vi "nirvimemoryEmulation.vi"(0 "Address":u32, 1 "Name":string, 2 "Depth":i32, 3 "Initialization Data":variant[](array[variant]), 5 "Data":i32, 7 "Write? (F)":bool, 9 "inTimedLoop":bool, 11 "error in":errorcluster, 12 "Local? (F)":bool, 13 "ref in wired":bool) -> (6 "Data":i32, 15 "error out":errorcluster)   [LabVIEW 2017]
uses:
  <vilib>/rvi/Emulation/niFpgaSctlEmulationSharedResMgrCmd.ctl
  <vilib>/rvi/Emulation/niFpgaSctlEmulationSharedResource.ctl
  <vilib>/rvi/Emulation/niFpgaSctlEmulationSharedResTypes.ctl
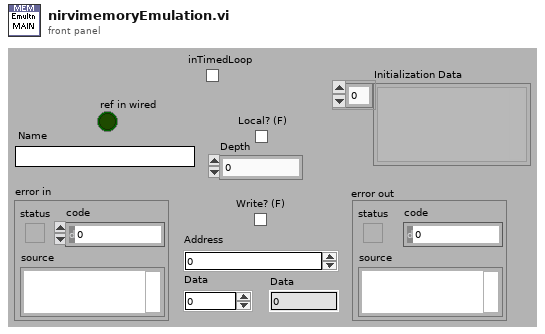
[diagram p1: front panel]
types:
  T1 = typedef "niFpgaSctlEmulationSharedResTypes.ctl" = enum16{"Global", "Register", "Fifo", "Full Memory", "Fast Memory", "Local"}
  T2 = typedef "niFpgaSctlEmulationSharedResource.ctl" = cluster{"resourceType":T1, "dataToWrite":variant, "ref":u32, "index":i32, "resourceName":string}
  T3 = typedef "niFpgaSctlEmulationSharedResMgrCmd.ctl" = enum16{"UpdateResources", "AddResource"}
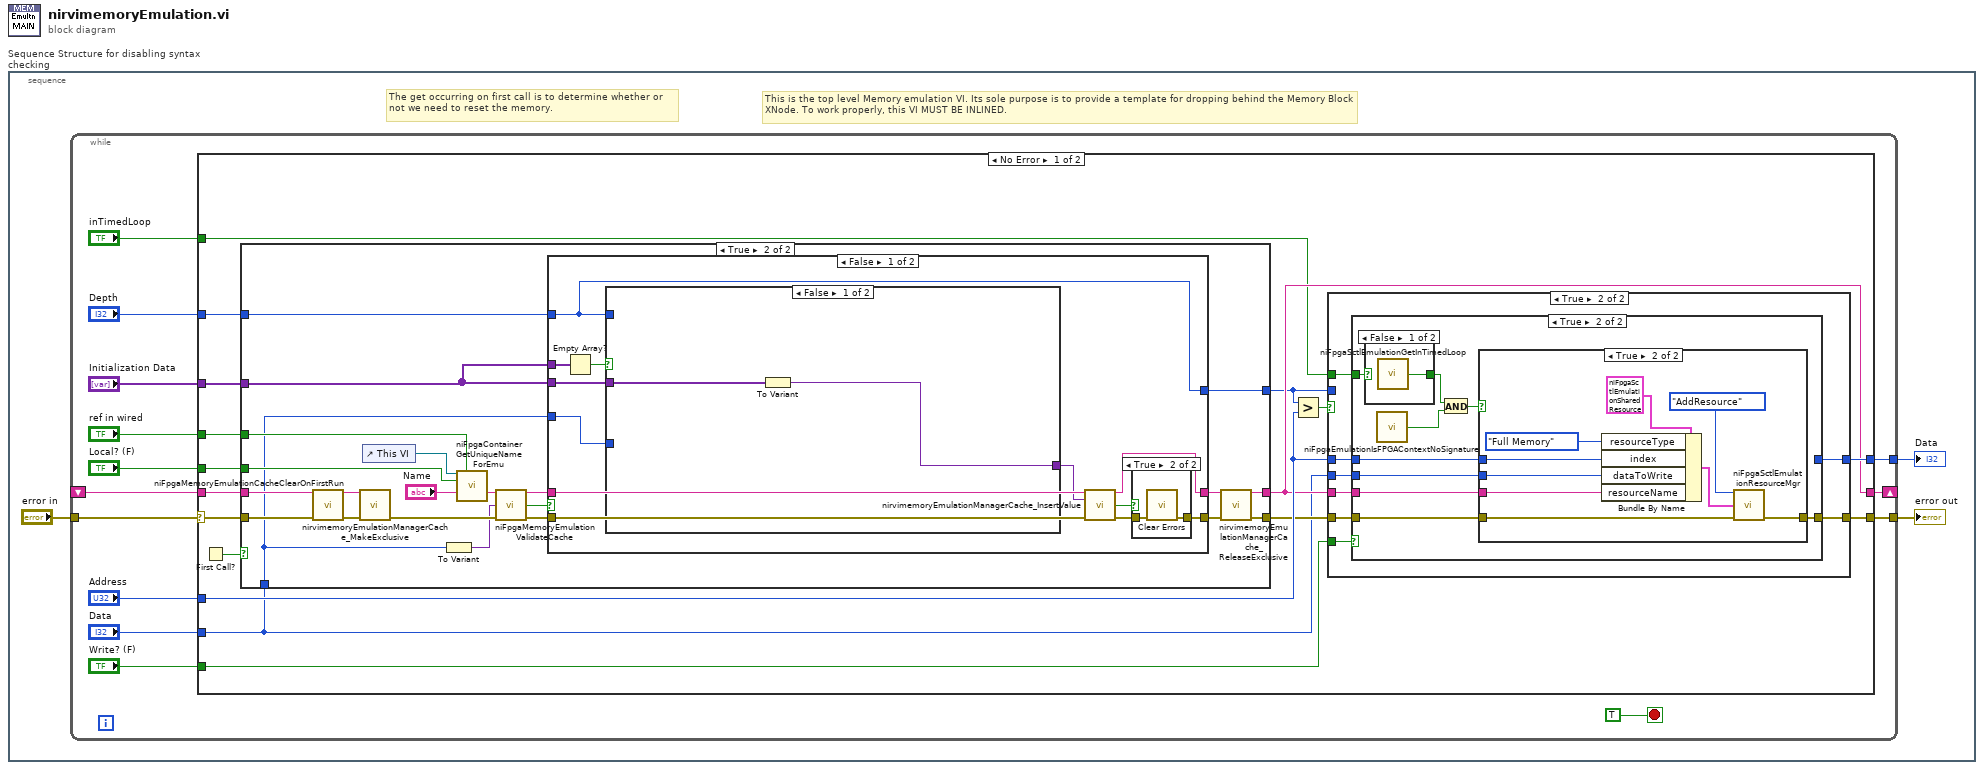
[diagram p0: block diagram]
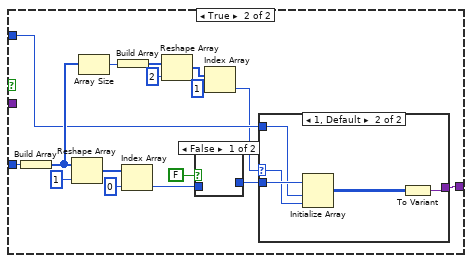
[diagram p3: hidden frame]
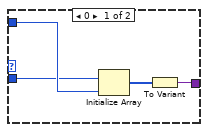
[diagram p4: hidden frame]
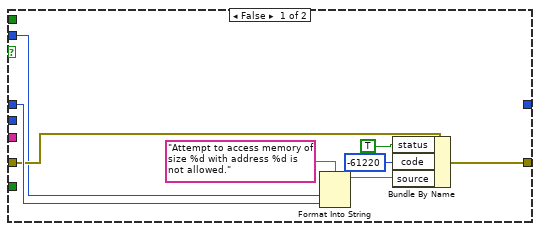
[diagram p8: hidden frame]
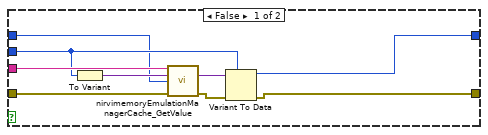
[diagram p9: hidden frame]
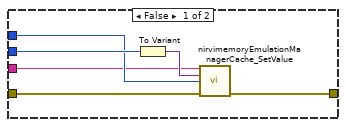
[diagram p11: hidden frame]
diagram:
  n1 = stacked-sequence "Sequence Structure for disabling syntax checking" {
    frame #0 {
      # "The get occurring on first call is to determine whether or not we need to reset the memory."
      # "This is the top level Memory emulation VI. Its sole purpose is to provide a template for dropping behind the Memory Block XNode. To work properly, this VI MUST BE INLINED."
      n2 = while {
        shift-right: [w15] -> _
        shift-left: _ -> [w17]
        tunnel: [w14] -> w1
        tunnel: [w13] -> w2
        tunnel: "error in" -> [w8]
        stop <- TRUE stop-if-true
        n3 = case shown="No Error" w8 {
          selector: w8 -> [w27 w158]
          tunnel: "Depth" -> [w25 _]
          tunnel: w17 -> [w26 w157]
          tunnel: [w29 w157] -> w15
          tunnel: "Write? (F)" -> [w32 _]
          tunnel: [w31 w158] -> w14
          tunnel: "Address" -> [w33 _]
          tunnel: "Data" -> [w24 _]
          tunnel: [w30 _] -> w13
          tunnel: "ref in wired" -> [w23 _]
          tunnel: "Local? (F)" -> [w22 _]
          tunnel: "inTimedLoop" -> [w19 _]
          tunnel: "Initialization Data" -> [w18 _]
          frame No Error {
            n4 = First Call?() -> (First Call?: T/F=w20:bool)
            n5 = case shown="True" w20 {
              tunnel: [w37 w59] -> w29
              tunnel: [w36 w58] -> w28
              tunnel: w27 -> [w36 w56]
              tunnel: w26 -> [w37 w55]
              tunnel: w25 -> [w35 w54]
              tunnel: w24 -> [_ w39]
              tunnel: w23 -> [_ w53]
              tunnel: w22 -> [_ w52]
              tunnel: [w35 w51] -> w21
              tunnel: w18 -> [_ w38]
              frame False {
              }
              frame True {
                n6 = call <vilib>:"niFpgaMemoryEmulationCacheClearOnFirstRun.vi"("Key"=w55, "error in"=w56) -> ("Key (dup)"=w50:string, "error out"=w57:errorcluster)  [unwired: 12 in]
                n7 = call <vilib>:"nirvimemoryEmulationManagerCache_MakeExclusive.vi"("Key"=w50, "error in"=w57) -> ("error out"=w41:errorcluster)  [unwired: 12 in, 1 out]
                n8 = control-ref of="This VI"() -> (w42:refnum<vi>)
                n9 = To Variant(anything=w39) -> (Variant=w40:variant)
                n10 = call <vilib>:"niFpgaContainerGetUniqueNameForEmu.vi"("parent VI"=w42, "ref in wired"=w53, "local"=w52, "name in"="Name") -> ("name out"=w44:string)  [unwired: 11 in]
                n11 = call <vilib>:"niFpgaMemoryEmulationValidateCache.vi"("key"=w44, "Data In"=w40, "error in"=w41) -> ("key (dup)"=w49:string, "found?"=w47:bool, "error out"=w48:errorcluster)  [unwired: 10 in]
                n12 = case shown="False" w47 {
                  tunnel: [w69 w105] -> w46
                  tunnel: [w60 w104] -> w51
                  tunnel: [w68 w103] -> w45
                  tunnel: w54 -> [w60 w104]
                  tunnel: w49 -> [w66 w105]
                  tunnel: w48 -> [w67 w103]
                  tunnel: w38 -> [w63 _]
                  tunnel: w38 -> [w62 _]
                  tunnel: w39 -> [w61 _]
                  frame False {
                    n13 = Empty Array?(array=w63) -> (empty?=w65:bool)
                    n14 = case shown="False" w65 {
                      tunnel: [w72 w74] -> w64
                      tunnel: w62 -> [w73 _]
                      tunnel: w61 -> [_ w80]
                      tunnel: w60 -> [_ w77]
                      frame False {
                        n15 = To Variant(anything=w73) -> (Variant=w72:variant)
                      }
                      frame True {
                        n16 = Build Array(w80) -> (w89:i32[])
                        n17 = Reshape Array(w89, 1 ("dimension size")) -> (w81:i32[])
                        n18 = Array Size(array=w89) -> (size(s)=w88:i32)
                        n19 = Build Array(w88) -> (w86:i32[])
                        n20 = Index Array(array=w81, index=0) -> (element=w76:i32)
                        n21 = Reshape Array(w86, 2 ("dimension size")) -> (w84:i32[])
                        n22 = case shown="False" FALSE {
                          tunnel: w76 -> [_ w99]
                          tunnel: [_ w99] -> w79
                          frame False {
                          }
                          frame True {
                          }
                        }
                        n23 = Index Array(array=w84, index=1) -> (element=w75:i32)
                        n24 = case shown="1, Default" w75 {
                          selector: w75 -> [_ w94]
                          tunnel: w79 -> [w91 w97]
                          tunnel: w77 -> [w92 w95]
                          tunnel: [w93 w98] -> w74
                          frame 0 {
                            n25 = Initialize Array(w91, w92) -> (w90:i32[])
                            n26 = To Variant(anything=w90) -> (Variant=w93:variant)
                          }
                          frame 1, Default {
                            n27 = Initialize Array(w97, w95, w94) -> (w96:i32[][])
                            n28 = To Variant(anything=w96) -> (Variant=w98:variant)
                          }
                        }
                      }
                    }
                    n29 = call <vilib>:"nirvimemoryEmulationManagerCache_InsertValue.vi"("Key"=w66, "Value"=w64, "error in (no error)"=w67) -> ("Key"=w69:string, "Found"=w71:bool, "error out"=w70:errorcluster)  [unwired: 1 in, 9 out]
                    n30 = case shown="True" w71 {
                      tunnel: w70 -> [w100 w102]
                      tunnel: [w100 w101] -> w68
                      frame False {
                      }
                      frame True {
                        n31 = call <vilib>:"Clear Errors.vi"("error in (no error)"=w102) -> ("error out"=w101:errorcluster)  [unwired: 1 in, 5 out]
                      }
                    }
                  }
                  frame True {
                  }
                }
                n32 = call <vilib>:"nirvimemoryEmulationManagerCache_ReleaseExclusive.vi"("Key"=w46, "error in"=w45) -> ("Key (dup)"=w59:string, "error out"=w58:errorcluster)  [unwired: 12 in]
              }
            }
            n33 = Greater?(x=w21, y=w33) -> (0:w34:bool)
            n34 = case shown="True" w34 {
              tunnel: w24 -> [_ w116]
              tunnel: w33 -> [w113 w119]
              tunnel: w28 -> [w112 w117]
              tunnel: w29 -> [_ w118]
              tunnel: w32 -> [_ w115]
              tunnel: [w111 w121] -> w31
              tunnel: [_ w120] -> w30
              tunnel: w21 -> [w107 _]
              tunnel: w19 -> [_ w114]
              frame False {
                n35 = Format Into String(format string="Attempt to access memory of size %d with address %d is not allowed." ("error message (\"\")"), w107, w113) -> (resulting string=w108:string)  [unwired: 2 in, 1 out]
                n36 = Bundle By Name(cluster=w112, "status"=TRUE, "code"=-61220, "source"=w108) -> (w111:errorcluster)
              }
              frame True {
                n37 = case shown="True" w115 {
                  tunnel: [w130 w135] -> w121
                  tunnel: [w123 _] -> w120
                  tunnel: w119 -> [w122 w139]
                  tunnel: w118 -> [w127 w136]
                  tunnel: w117 -> [w126 w137]
                  tunnel: w116 -> [w124 w138]
                  tunnel: w114 -> [_ w134]
                  frame False {
                    n38 = To Variant(anything=w124) -> (Variant=w125:variant)
                    n39 = call <vilib>:"nirvimemoryEmulationManagerCache_GetValue.vi"("Key"=w127, "Value"=w125, "Address"=w122, "error in (no error)"=w126) -> ("Value"=w128:variant, "error out"=w129:errorcluster)  [unwired: 10 out]
                    n40 = Variant To Data(error in=w129, type=w124, Variant=w128) -> (data=w123:i32, error out=w130:errorcluster)
                  }
                  frame True {
                    n41 = case shown="False" w134 {
                      selector: w134 -> [_ w141]
                      tunnel: [w140 w141] -> w133
                      frame False {
                        n42 = call <vilib>:"niFpgaSctlEmulationGetInTimedLoop.vi"() -> ("x != 0?"=w140:bool)  [unwired: 15 in]
                      }
                      frame True {
                      }
                    }
                    n43 = call <vilib>:"niFpgaEmulationIsFPGAContextNoSignature.vi"() -> ("Is Fpga Context?"=w132:bool)  [unwired: 15 in]
                    n44 = And(x=w133, y=w132) -> (x .and. y?=w131:bool)
                    n45 = case shown="True" w131 {
                      tunnel: w139 -> [w145 w153]
                      tunnel: w138 -> [w147 w148]
                      tunnel: w137 -> [w143 w156]
                      tunnel: w136 -> [w144 w154]
                      tunnel: [w142 w155] -> w135
                      frame False {
                        n46 = To Variant(anything=w147) -> (Variant=w146:variant)
                        n47 = call <vilib>:"nirvimemoryEmulationManagerCache_SetValue.vi"("Key"=w144, "Value"=w146, "Address"=w145, "error in (no error)"=w143) -> ("error out"=w142:errorcluster)  [unwired: 11 out]
                      }
                      frame True {
                        n48 = Bundle By Name(cluster=T2 {"resourceType"=enum."Global", "dataToWrite"=variant, "ref"=0, "index"=0, "resourceName"="GlobalData.vi"} ("SharedResourceItem"), "resourceType"=niFpgaSctlEmulationSharedResTypes."Full Memory", "index"=w153, "dataToWrite"=w148, "resourceName"=w154) -> (w150:T2)
                        n49 = call <vilib>:"niFpgaSctlEmulationResourceMgr.vi"("Command"=niFpgaSctlEmulationSharedResMgrCmd."AddResource", "SharedResourceItem"=w150, "error in"=w156) -> ("error out"=w155:errorcluster)  [unwired: 12 in]
                      }
                    }
                  }
                }
              }
            }
          }
          frame Error {
          }
        }
      }
      "error out" <- w1
      "Data" <- w2
    }
  }
